vi "to_json.vi"(8 "error in":errorcluster, 11 "exclude in":refnum<class "exclude.lvclass">) -> (0 "error out":errorcluster, 2 "json":string, 3 "exclude out":refnum<class "exclude.lvclass">)   [LabVIEW 2020, in "nominal types.lvlib" / "channelFilter.lvlib" / "exclude.lvclass"]
uses:
  exclude.lvclass
  exclude.lvclass/exclude.ctl
  d2a2ac13-5471-4191-9e88-4f0084fe2bd1.vi
  <vilib>/JDP Science/JSONtext/support/Format JSON Array Text.vi
  <vilib>/JDP Science/JSONtext/Variant to JSON Text.vi
  <vilib>/JDP Science/JSONtext/support/Format JSON Object.vi
  <vilib>/JDP Science/JSONtext/LVClass Serializer/JSONtext LVClass Serializer.lvclass
  <vilib>/JDP Science/JSONtext/JSONtext.lvlib
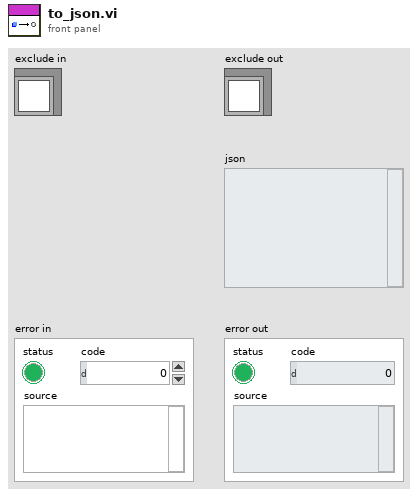
[diagram p1: front panel]
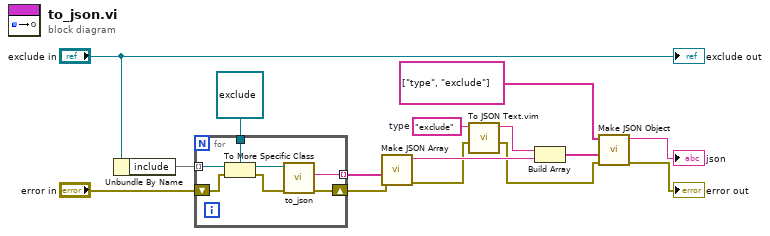
[diagram p0: block diagram]
diagram:
  w9 = "exclude"  # type
  n1 = Unbundle By Name("exclude in") -> ("include"=w14:set{refnum<class>})
  n2 = for {
    tunnel: w14 -> [w22] mode=indexing
    tunnel: refnum<class "exclude.lvclass"> refnum ("nominal types.lvlib:channelFilter.lvlib:include.lvclass") -> [w21]
    tunnel: [w19] -> w11 mode=indexing
    shift-right: [w17] -> w10
    shift-left: "error in" -> [w16]
    n3 = To More Specific Class(target class=w21, reference=w22, error in=w16) -> (specific class reference=w20:refnum<class "exclude.lvclass">, error out=w18:errorcluster)
    n4 = call-dynamic "to_json.vi"("error in"=w18, "exclude in"=w20) -> ("error out"=w17:errorcluster, "json"=w19:string)  [unwired: 7 in, 1 out]
  }
  n5 = call <vilib>:"Make JSON Array.vi"("error in (no error)"=w10, "JSON Elements"=w11) -> ("error out"=w6:errorcluster, "<JSON>"=w7:string)  [unwired: 8 in]
  n6 = call "To JSON Text.vim"("error in (no error)"=w6, "Anything"=w9) -> ("error out"=w3:errorcluster, "<JSON>"=w8:string)  [unwired: 8 in]
  n7 = Build Array(w8, w7) -> (w5:string[])
  n8 = call <vilib>:"Make JSON Object.vi"("error in (no error)"=w3, "JSON Items"=w5, "Item Names"=string[] ["type", "exclude"]) -> ("error out"=→"error out":errorcluster, "<JSON>"=→"json":string)  [unwired: 7 in]
  "exclude out" <- "exclude in"
